vi "Start_Pos_Case_Structures_r0.vi"() -> ()   [LabVIEW 2015]
panel:
  out "Angle":dbl
  out "Goal":dbl
  in  "Angle":dbl
  in  "Y Start":dbl
  in  "X Start":dbl
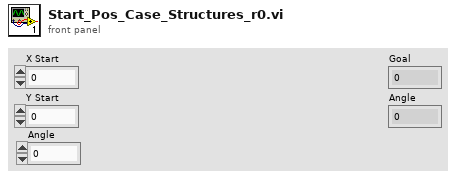
[diagram p1: front panel]
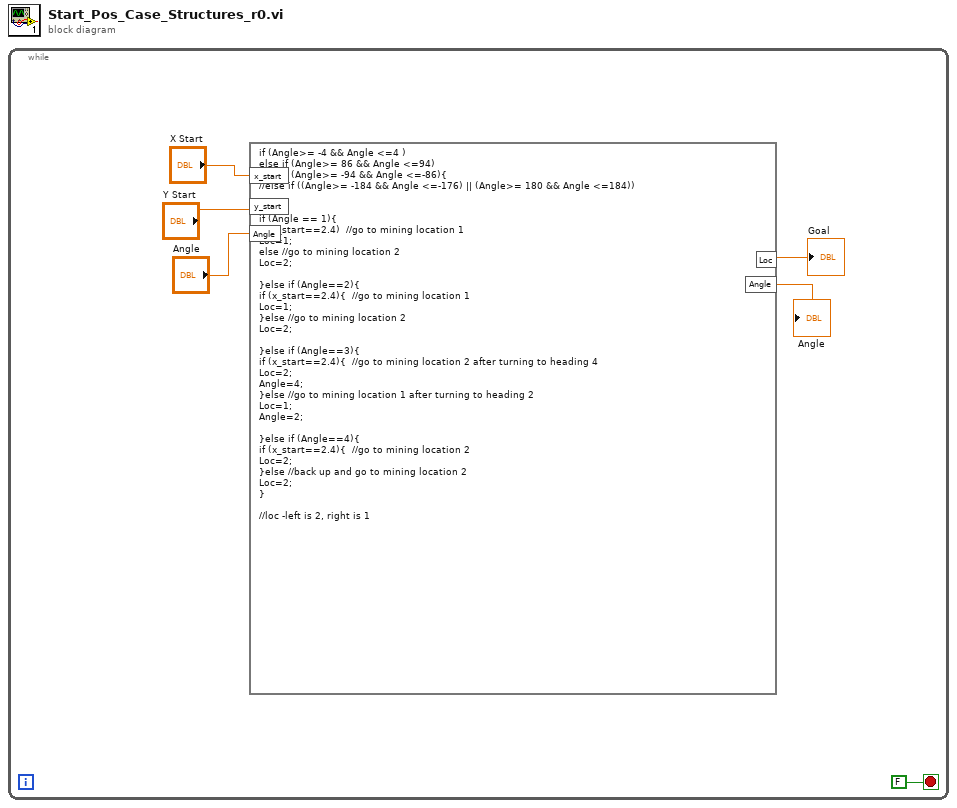
[diagram p0: block diagram]
diagram:
  n1 = while {
    stop <- FALSE stop-if-true
    n2 = formula code="if (Angle>= -4 && Angle <=4 )\nelse if (Angle>= 86 && Angle <=94)\nelse if (Angle>= -94 && Angle <=-86){\n//else if ((Angle>= -184 && Angle <=-176) || (Angle>= 180 && Angle <=184))\n\n\nif (Angle == 1){\nif (x_start==2.4)  //go to mining location 1\nLoc=1;\nelse //go to mining location 2\nLoc=2;\n\n}else if (Angle==2){\nif (x_start==2.4){  //go to mining location 1\nLoc=1;\n}else //go to mining location 2\nLoc=2;\n\n}else if (Angle==3){\nif (x_start==2.4){  //go to mining location 2 after turning to heading 4\nLoc=2;\nAngle=4;\n}else //go to mining location 1 after turning to heading 2\nLoc=1;\nAngle=2;\n\n}else if (Angle==4){\nif (x_start==2.4){  //go to mining location 2\nLoc=2;\n}else //back up and go to mining location 2\nLoc=2;\n}\n\n//loc -left is 2, right is 1"("x_start"="X Start", "y_start"="Y Start", "Angle"="Angle") -> ("Loc"=→"Goal":dbl, "Angle"=→"Angle":dbl)
  }
